vi "CalibArrData.vi"() -> ()   [LabVIEW 2014]
panel:
  in  "Size":cluster{"X":dbl, "Y":dbl}
  in  "BoardPts(A)":cluster{dbl, dbl}[][](array[cluster])
  in  "RBPTS(B)":cluster{sgl, sgl}[][](array[cluster])
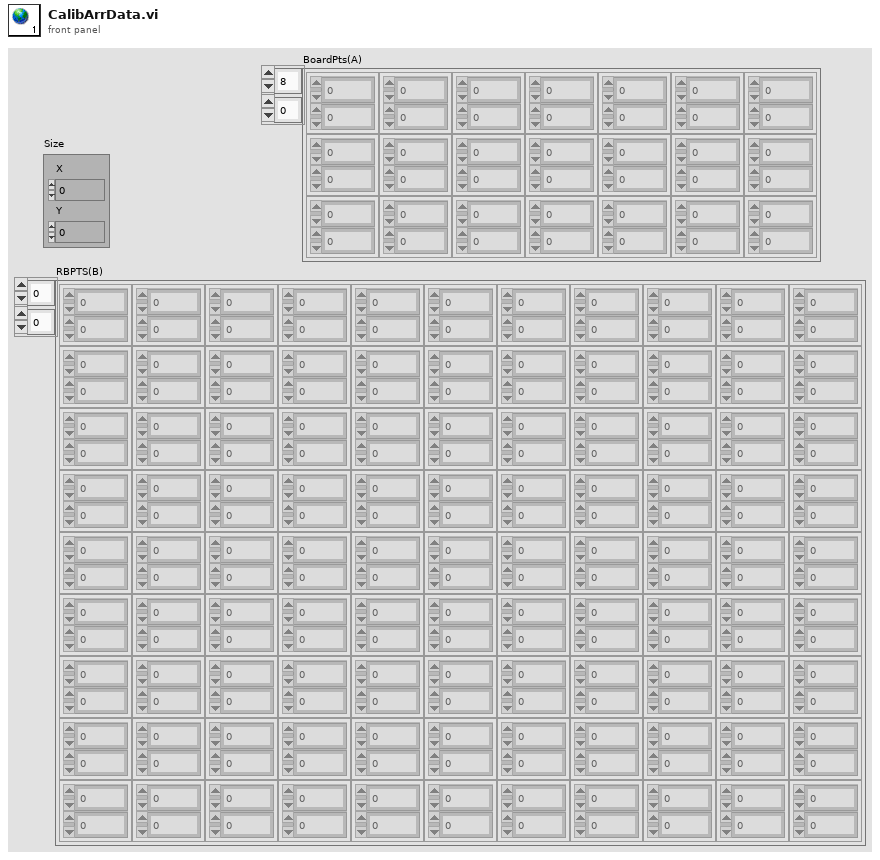
[diagram p1: front panel]
diagram:
